vi "Icon.vi"(8 "error in (no error)":errorcluster, 11 "Device in":refnum<class "Device.lvclass">) -> (0 "error out":errorcluster, 2 "Icon":T1, 3 "Device out":refnum<class "Device.lvclass">)   [LabVIEW 2015, in "IBEX Device.lvlib" / "Device.lvclass"]
doc: "Provides a 16x16 pixel icon for the device."
uses:
  Device.lvclass
  <vilib>/picture/picture.llb/imagedata.ctl
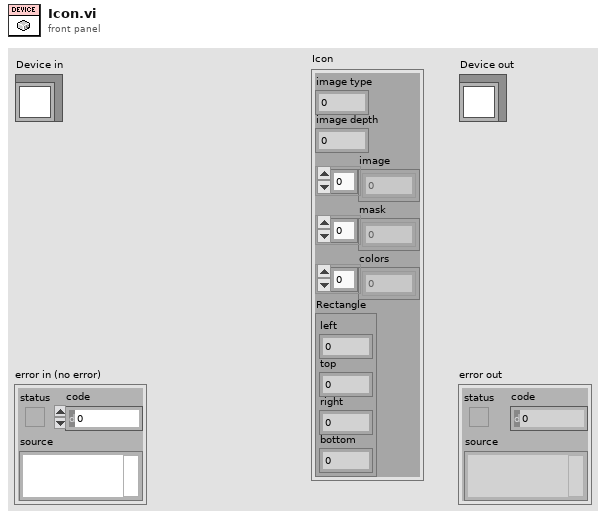
[diagram p1: front panel]
types:
  T1 = typedef "imagedata.ctl" = cluster{"image type":i32, "image depth":i32, "image":u8[], "mask":u8[], "colors":u32[], "Rectangle":cluster{"left":i16, "top":i16, "right":i16, "bottom":i16}}
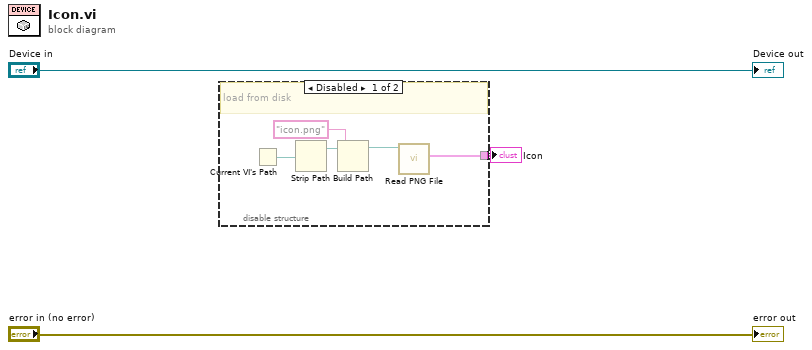
[diagram p0: block diagram]
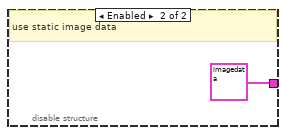
[diagram p2: hidden frame]
diagram:
  n1 = disable-structure shown="Disabled" {
    disable-tunnel: [w4 T1 {"image type"=0, "image depth"=32, "image"=array[1024 elements], "mask"=[0, 0, 0, 0, 0, 0, 1, 192, 7, 240, 31, 252, 39, 242, 57, 206, 62, 190, 63, 126, 63, 126, 31, 124, 7, 112, 1, 192, 0, 0, 0, 0], "colors"=[], "Rectangle"={"left"=0, "top"=0, "right"=16, "bottom"=16}} ("image data")] -> w1
    frame Disabled {
      # "load from disk"
      n2 = Current VI's Path() -> (path=w7:path)
      n3 = Strip Path(path=w7) -> (stripped path=w8:path)  [unwired: 1 out]
      n4 = Build Path(base path=w8, name or relative path="icon.png") -> (appended path=w6:path)
      n5 = call <vilib>:"Read PNG File.vi"("path to PNG file"=w6) -> ("image data"=w4:T1)  [unwired: 8 in, 2 out]
    }
    frame Enabled {
      # "use static image data"
    }
  }
  "Icon" <- w1
  "error out" <- "error in (no error)"
  "Device out" <- "Device in"
